vi "SP_BusyCheck.vi"(8 "error in (no error)":errorcluster, 11 "SemiProbe in":refnum<class "SemiProbe.lvclass">) -> (0 "error out":errorcluster, 3 "SemiProbe out":refnum<class "SemiProbe.lvclass">)   [LabVIEW 2013, in "SemiProbe.lvclass"]
uses:
  SemiProbe.lvclass
  SP_Exchange.vi
panel:
  in  "stop":bool
  out "SemiProbe Busy":bool
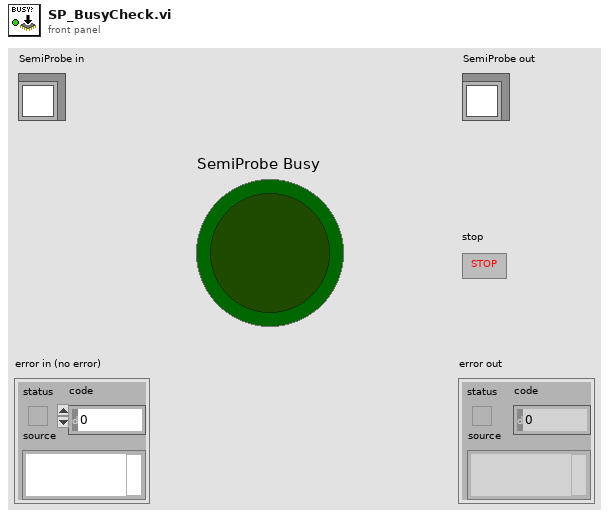
[diagram p1: front panel]
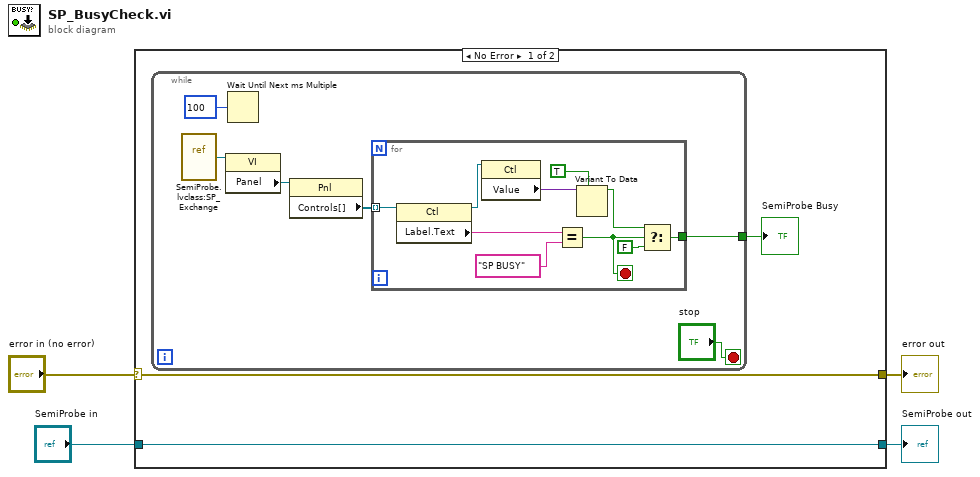
[diagram p0: block diagram]
diagram:
  n1 = case shown="No Error" "error in (no error)" {
    selector: "error in (no error)" -> [w6 w25]
    tunnel: [w6 w25] -> w3
    tunnel: [w7 w24] -> w1
    tunnel: "SemiProbe in" -> [w7 w24]
    frame No Error {
      n2 = while {
        tunnel: [w9] -> w5
        stop <- "stop" stop-if-true
        n3 = vi-ref "SemiProbe.lvclass:SP_Exchange.vi"() -> (w12:refnum<vi>)
        n4 = property class="VI"(reference=w12) -> ("Panel"=w11:refnum<vi>)  [unwired: 1 in, 2 out]
        n5 = Wait Until Next ms Multiple(millisecond multiple=100) -> ()  [unwired: 1 out]
        n6 = property class="Pnl"(reference=w11) -> ("Controls[]"=w10:refnum<vi>[])  [unwired: 1 in, 2 out]
        n7 = for {
          tunnel: w10 -> [w23] mode=indexing
          tunnel: [w16] -> w9
          stop <- w14 stop-if-true
          n8 = property class="Ctl"(reference=w23) -> (reference out=w22:refnum<vi>, "Label.Text"=w19:string)  [unwired: 1 in, 1 out]
          n9 = property class="Ctl"(reference=w22) -> ("Value"=w20:variant)  [unwired: 1 in, 2 out]
          n10 = Equal?(x=w19, y="SP BUSY") -> (x = y?=w14:bool)
          n11 = Variant To Data(type=TRUE, Variant=w20) -> (data=w17:bool)  [unwired: 1 in, 1 out]
          n12 = Select(t=w17, s=w14, f=FALSE) -> (s? t:f=w16:bool)
        }
      }
      "SemiProbe Busy" <- w5
    }
    frame Error {
    }
  }
  "error out" <- w3
  "SemiProbe out" <- w1
